vi "Configure Scan Layer Trigger Source.vi"(6 "Scan Timer Interval (0.1)":dbl=0.1 format="%#.6g", 7 "Scan Delay (0 s)":dbl format="%#.6g", 8 "error in (no error)":errorcluster, 9 "Scan Count (1)":i32=1, 10 "Scan Source (1: Immediate)":i32(ring)=1 items=["Hold"=0, "Immediate"=1, "Manual"=3, "Bus"=4, "Trigger Link"=5, "External Triggering"=6, "Timer "=7], 11 "VISA resource name":refnum<visa-resource-name>) -> (0 "error out":errorcluster, 3 "VISA resource name out":refnum<visa-resource-name>)   [LabVIEW 2020, in "Keithley 6517.lvlib"]
doc: "Configures the source, count, delay and time interval for the Scan Layer (Arm2) of the trigger model.\n\n<B>Note:</B>\n(1)<B>Models 6517A, 6517B:</B> The trigger model consists of 3 layers, the Arm Layer, the Scan Layer (Arm2), and the Measure Layer (Trigger).\n(2)<B>Model 6514:</B> The trigger model consists of 2 layers: Arm Layer & Measure Layer (Trigger).\n\nThis VI is <B>NOT</B> compatible with model <B>6514</B>."
uses:
  <instrlib>/Keithley 6517/Keithley 6517.lvlib
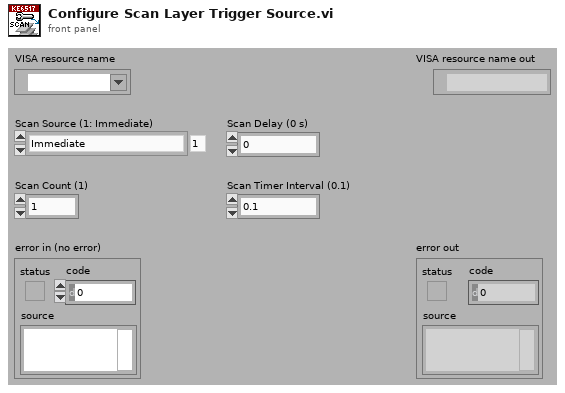
[diagram p1: front panel]
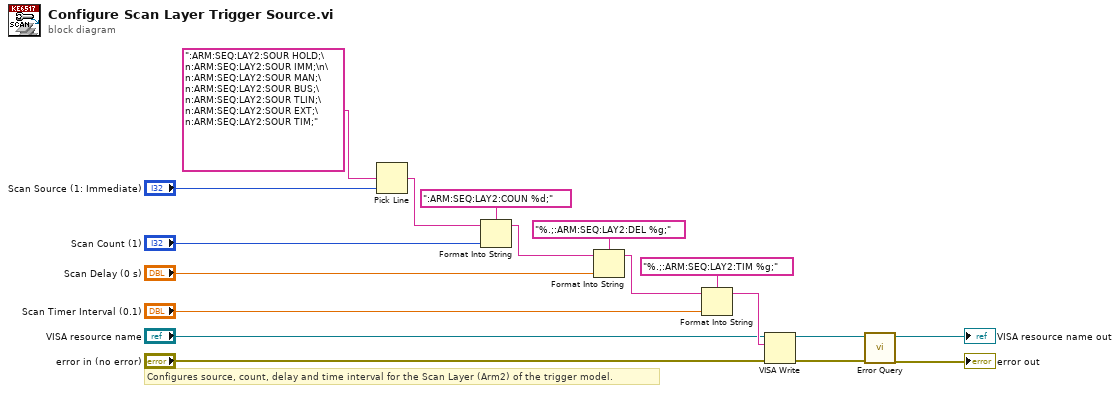
[diagram p0: block diagram]
diagram:
  # "Configures source, count, delay and time interval for the Scan Layer (Arm2) of the trigger model."
  n1 = Pick Line(multi-line string=":ARM:SEQ:LAY2:SOUR HOLD;\n:ARM:SEQ:LAY2:SOUR IMM;\n\n:ARM:SEQ:LAY2:SOUR MAN;\n:ARM:SEQ:LAY2:SOUR BUS;\n:ARM:SEQ:LAY2:SOUR TLIN;\n:ARM:SEQ:LAY2:SOUR EXT;\n:ARM:SEQ:LAY2:SOUR TIM;", line index="Scan Source (1: Immediate)") -> (output string=w2:string)  [unwired: 1 in]
  n2 = Format Into String(format string=":ARM:SEQ:LAY2:COUN %d;", initial string=w2, "Scan Count (1)") -> (resulting string=w16:string)  [unwired: 1 in, 1 out]
  n3 = Format Into String(format string="%.;:ARM:SEQ:LAY2:DEL %g;", initial string=w16, "Scan Delay (0 s)") -> (resulting string=w1:string)  [unwired: 1 in, 1 out]
  n4 = Format Into String(format string="%.;:ARM:SEQ:LAY2:TIM %g;", initial string=w1, "Scan Timer Interval (0.1)") -> (resulting string=w11:string)  [unwired: 1 in, 1 out]
  n5 = VISA Write(VISA resource name="VISA resource name", write buffer=w11, error in (no error)="error in (no error)") -> (VISA resource name out=w8:refnum<visa-resource-name>, error out=w7:errorcluster)  [unwired: 1 out]
  n6 = call <instrlib>:"Error Query.vi"("error in (no error)"=w7, "VISA resource name"=w8) -> ("error out"=→"error out":errorcluster, "VISA resource name out"=→"VISA resource name out":refnum<visa-resource-name>)  [unwired: 6 in, 2 out]
